vi "serial_connection_FSM.vi"(0 "commands_q":refnum<queue>, 5 "sensor_data_q":refnum<queue>, 11 "error in (no error)":errorcluster) -> (15 "error out":errorcluster)   [LabVIEW 2019]
uses:
  arduino_FSM.ctl
  <vilib>/Instr/_visa.llb/VISA Configure Serial Port (Instr).vi
panel:
  out "read buffer":string
  in  "VISA resource name out":refnum<visa-resource-name>
  out "Sampling Frequency":string
  out "COM port":string="COM5"
  out "baud RATE":string="9600"
  in  "state_and_args":string
  out "Arduino FSM":T1
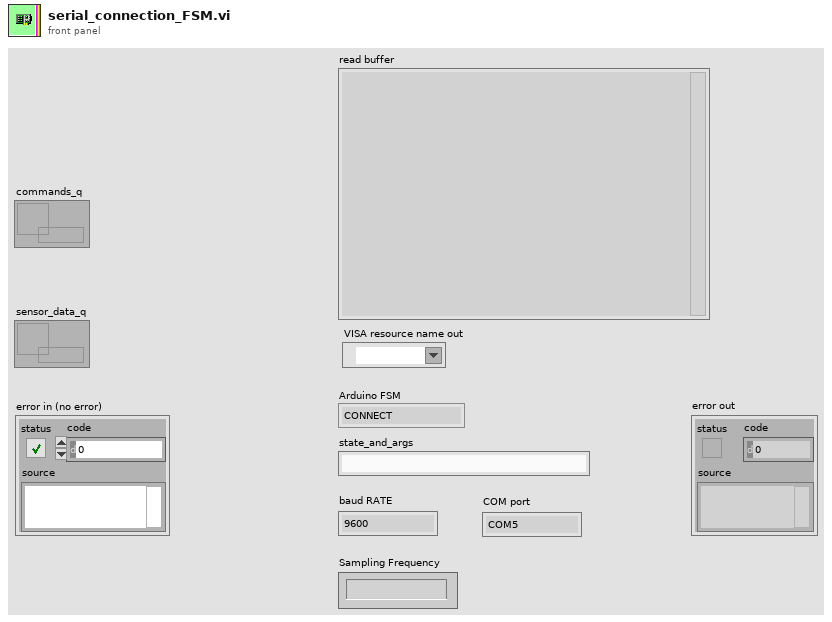
[diagram p1: front panel]
types:
  T1 = typedef "arduino_FSM.ctl" = enum16{"CONNECT", "WAITING", "DISCONNECT", "READ", "WRITE", "WRONG_OP", "BYTE AVAIL?"}
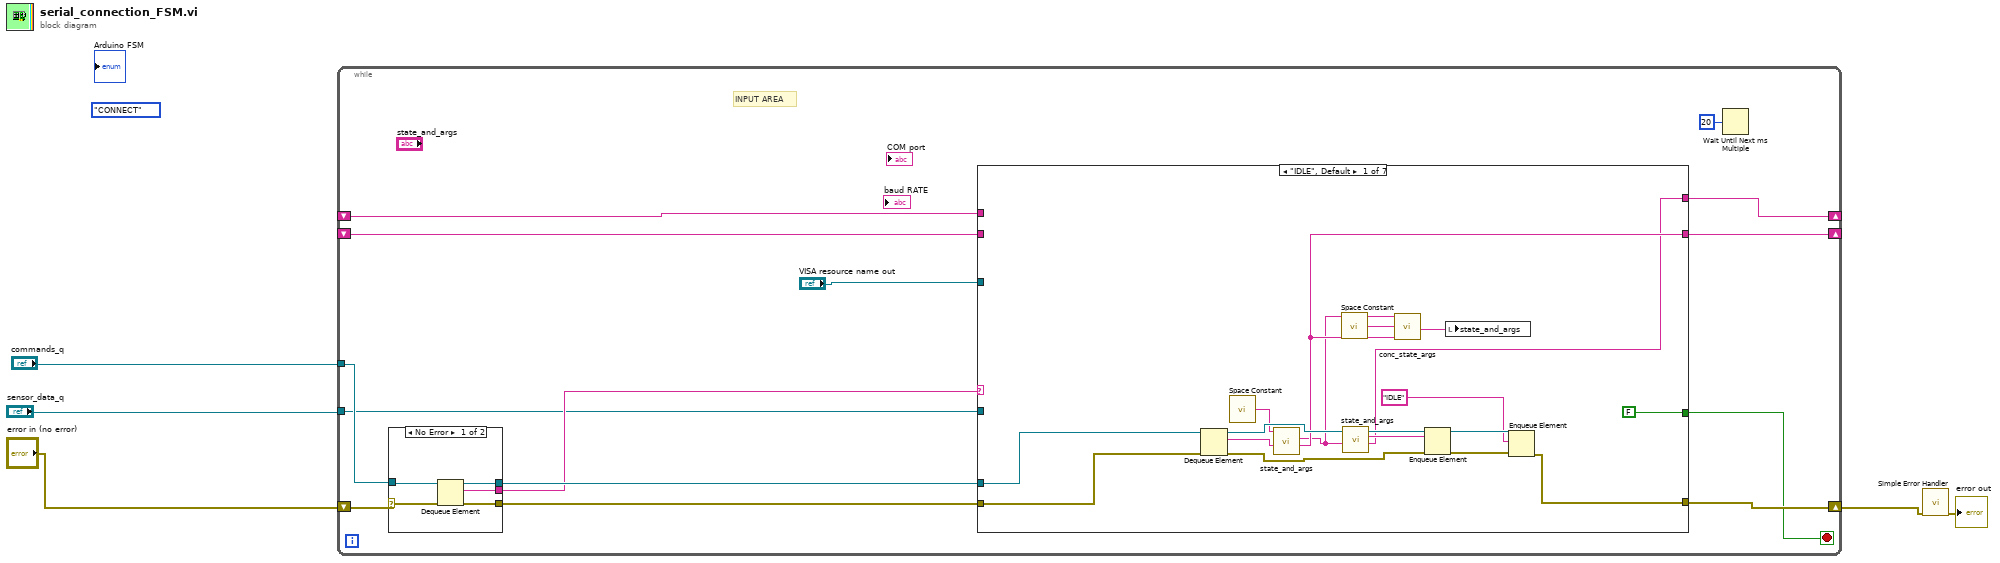
[diagram p0: block diagram]
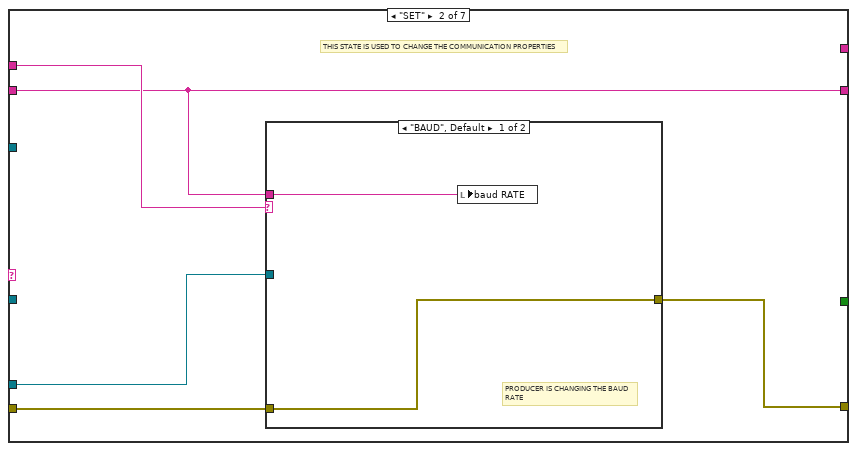
[diagram p2: hidden frame]
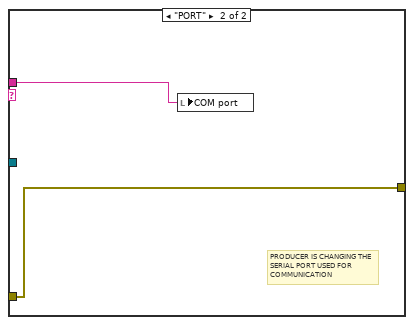
[diagram p3: hidden frame]
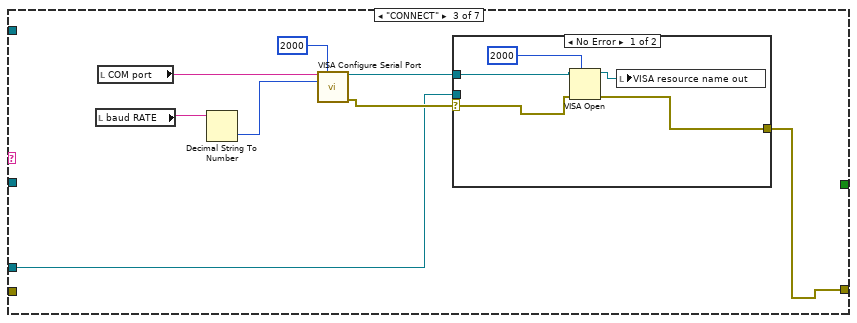
[diagram p4: hidden frame]
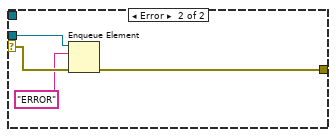
[diagram p5: hidden frame]
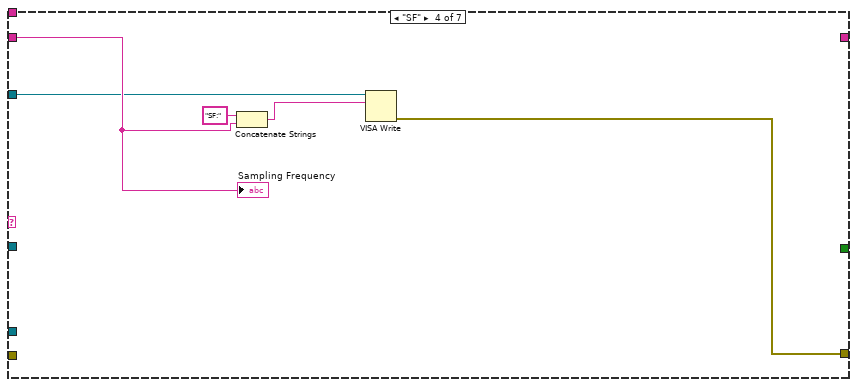
[diagram p6: hidden frame]
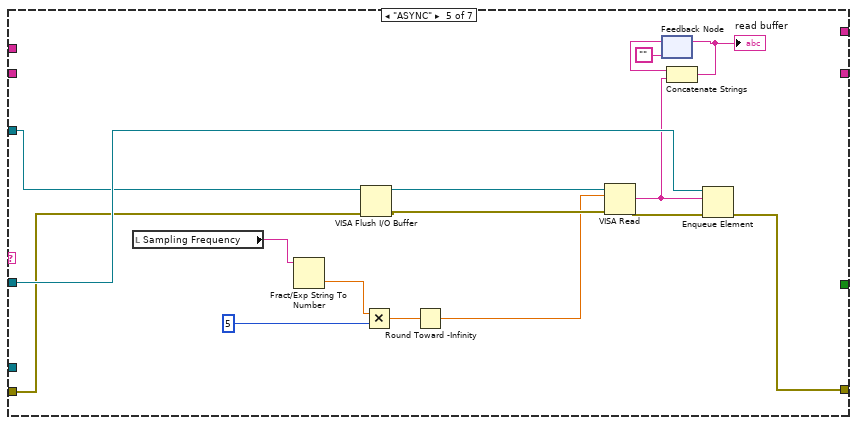
[diagram p7: hidden frame]
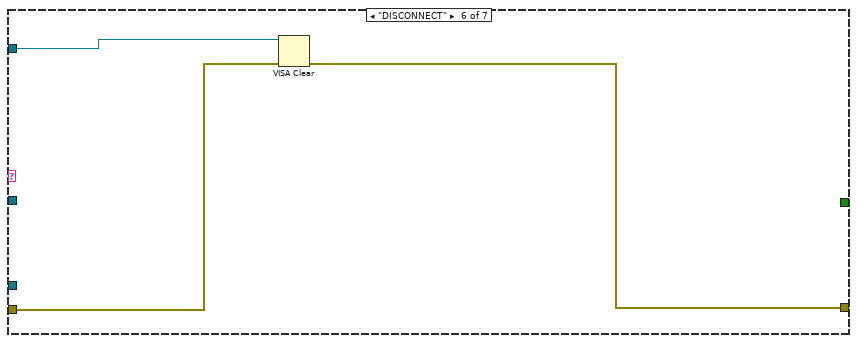
[diagram p8: hidden frame]
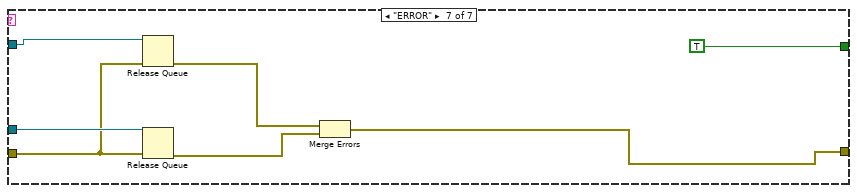
[diagram p9: hidden frame]
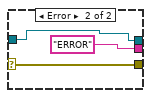
[diagram p10: hidden frame]
diagram:
  (unwired) arduino_FSM."CONNECT" ("Arduino FSM")
  n1 = while {
    tunnel: "commands_q" -> [w18]
    shift-right: [w12] -> w4
    shift-left: "error in (no error)" -> [w19]
    shift-right: [w13] -> _
    shift-left: _ -> [w14]
    tunnel: "sensor_data_q" -> [w11]
    shift-right: [w8] -> _
    shift-left: _ -> [w7]
    stop <- w10 stop-if-true
    # "INPUT AREA"
    n2 = case shown="No Error" w19 {
      selector: w19 -> [w98 w99]
      tunnel: w18 -> [w97 w100]
      tunnel: [w96 w100] -> w17
      tunnel: [w95 w99] -> w16
      tunnel: [w94 "ERROR"] -> w15
      frame No Error {
        n3 = Dequeue Element(queue=w97, error in (no error)=w98) -> (queue out=w96:refnum<queue>, element=w94:string, error out=w95:errorcluster)  [unwired: 1 in, 1 out]
      }
      frame Error {
      }
    }
    n4 = case shown="\"IDLE\", Default" w15 {
      tunnel: w17 -> [w35 w41 w47 _ _ _ w92]
      tunnel: w16 -> [w34 w40 _ _ w69 w86 w91]
      tunnel: w14 -> [_ w37 _ w64 _ _ _]
      tunnel: [w27 w37 _ _ _ _ _] -> w13
      tunnel: [w28 w39 w46 w65 w77 w85 w88] -> w12
      tunnel: w11 -> [_ _ _ _ w79 _ w93]
      tunnel: [FALSE _ _ _ _ _ TRUE] -> w10
      tunnel: [w20 _ _ _ _ _ _] -> w8
      tunnel: w7 -> [_ w38 _ _ _ _ _]
      tunnel: "VISA resource name out" -> [_ _ _ w63 w72 w84 _]
      frame "IDLE", Default {
        n5 = Dequeue Element(queue=w35, error in (no error)=w34) -> (queue out=w32:refnum<queue>, element=w33:string, error out=w23:errorcluster)  [unwired: 1 in, 1 out]
        n6 = call <vilib>:"Space Constant.vi"() -> ("String"=w24:string)
        n7 = call "state_and_args.vi"("String"=w33, "DELIMITER (:)"=w24) -> ("Arguments"=w27:string, "State"=w22:string)  [unwired: 8 in]
        n8 = call <vilib>:"Space Constant.vi"() -> ("String"=w25:string)
        n9 = call "state_and_args.vi"("String"=w22) -> ("Arguments"=w20:string, "State"=w21:string)  [unwired: 9 in]
        n10 = call "conc_state_args.vi"("State"=w22, "DELIMITER (:)"=w25, "Args"=w27) -> ("state_and_args"=w26:string)  [unwired: 12 in]
        n11 = Enqueue Element(queue=w32, element=w21, error in (no error)=w23) -> (queue out=w31:refnum<queue>, error out=w30:errorcluster)  [unwired: 1 in, 1 out]
        n12 = local write "state_and_args"(w26) -> ()
        n13 = Enqueue Element(queue=w31, element="IDLE", error in (no error)=w30) -> (error out=w28:errorcluster)  [unwired: 1 in, 2 out]
      }
      frame "SET" {
        # "THIS STATE IS USED TO CHANGE THE COMMUNICATION PROPERTIES"
        n14 = case shown="\"BAUD\", Default" w38 {
          tunnel: w41 -> [_ _]
          tunnel: w40 -> [w43 w45]
          tunnel: [w43 w45] -> w39
          tunnel: w37 -> [w42 w44]
          frame "BAUD", Default {
            # "PRODUCER IS CHANGING THE BAUD\nRATE"
            n15 = local write "baud RATE"(w42) -> ()
          }
          frame "PORT" {
            # "PRODUCER IS CHANGING THE\nSERIAL PORT USED FOR \nCOMMUNICATION"
            n16 = local write "COM port"(w44) -> ()
          }
        }
      }
      frame "CONNECT" {
        n17 = local read "baud RATE"() -> (w52:string)
        n18 = local read "COM port"() -> (w53:string)
        n19 = Decimal String To Number(string=w52) -> (number=w51:i32)  [unwired: 2 in, 1 out]
        n20 = call-poly "VISA Configure Serial Port"("VISA resource name"=w53, "timeout (10sec)"=u32 2000, "baud rate (9600)"=w51) -> ("VISA resource name out"=w49:refnum<visa-resource-name>, "error out"=w48:errorcluster)  [unwired: 11 in]
        n21 = case shown="No Error" w48 {
          selector: w48 -> [w57 w62]
          tunnel: w49 -> [w58 _]
          tunnel: w47 -> [_ w61]
          tunnel: [w56 w59] -> w46
          frame No Error {
            n22 = VISA Open(timeout (0)=u32 2000 ("VISA Open timeout (0)"), error in (no error)=w57, VISA resource name=w58) -> (VISA resource name=w54:refnum<visa-resource-name>, error out=w56:errorcluster)  [unwired: 2 in]
            n23 = local write "VISA resource name out"(w54) -> ()
          }
          frame Error {
            n24 = Enqueue Element(queue=w61, element="ERROR", error in (no error)=w62) -> (error out=w59:errorcluster)  [unwired: 1 in, 2 out]
          }
        }
      }
      frame "SF" {
        n25 = Concatenate Strings("SF:" ("string"), w64) -> (w66:string)
        n26 = VISA Write(VISA resource name=w63, write buffer=w66) -> (error out=w65:errorcluster)  [unwired: 1 in, 2 out]
        "Sampling Frequency" <- w64
      }
      frame "ASYNC" {
        n27 = local read "Sampling Frequency"() -> (w83:string)
        n28 = Fract/Exp String To Number(string=w83) -> (number=w82:dbl)  [unwired: 3 in, 1 out]
        n29 = VISA Flush I/O Buffer(VISA resource name=w72, error in (no error)=w69) -> (VISA resource name out=w71:refnum<visa-resource-name>, error out=w70:errorcluster)  [unwired: 1 in]
        n30 = Multiply(x=w82, y=5) -> (x*y=w80:dbl)
        n31 = Round Toward -Infinity(1:w80) -> (0:w68:dbl)
        n32 = VISA Read(VISA resource name=w71, byte count=w68, error in (no error)=w70) -> (read buffer=w73:string, error out=w78:errorcluster)  [unwired: 2 out]
        n33 = feedback #1("") -> (w76:string)
        n34 = Concatenate Strings(w76, w73) -> (w74:string)
        "read buffer" <- w74
        n35 = feedback-in #1(w74) -> ()
        n36 = Enqueue Element(queue=w79, element=w73, error in (no error)=w78) -> (error out=w77:errorcluster)  [unwired: 1 in, 2 out]
      }
      frame "DISCONNECT" {
        n37 = VISA Clear(VISA resource name=w84, error in (no error)=w86) -> (error out=w85:errorcluster)  [unwired: 1 out]
      }
      frame "ERROR" {
        n38 = Release Queue(queue=w93, error in (no error)=w91) -> (error out=w90:errorcluster)  [unwired: 1 in, 2 out]
        n39 = Release Queue(queue=w92, error in (no error)=w91) -> (error out=w89:errorcluster)  [unwired: 1 in, 2 out]
        n40 = Merge Errors(w90, w89) -> (w88:errorcluster)
      }
    }
    n41 = Wait Until Next ms Multiple(millisecond multiple=u32 20) -> ()  [unwired: 1 out]
  }
  n42 = call <vilib>:"Simple Error Handler.vi"("error in (no error)"=w4) -> ("error out"=→"error out":errorcluster)  [unwired: 4 in, 4 out]
